vi "gemm - General Matrix-Matrix Product.vi"   [LabVIEW 2020, in "NI_AALBLAS.lvlib"]
doc: "Calculates the product of two general matrices."
uses:
  NI_AALBLAS.lvlib
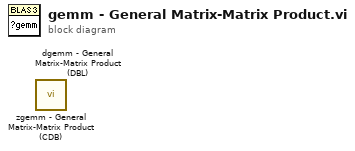
[diagram p0: block diagram]
diagram:
  n1 = call "zgemm - General Matrix-Matrix Product (CDB).vi"() -> ()  [unwired: 10 in, 2 out]
  n2 = call "dgemm - General Matrix-Matrix Product (DBL).vi"() -> ()  [unwired: 10 in, 2 out]
